vi "CheckListener ConvBox.vi"(8 "error in":errorcluster, 9 "address string":string, 11 "VISA resource in":refnum<visa-resource-name>) -> (0 "error out":errorcluster, 1 "listener found":bool, 2 "ibsta":T1, 3 "VISA resource out":refnum<visa-resource-name>)   [LabVIEW 2019, in "Protocols.lvlib" / "RS-xxx to GPIB ConvBox.lvclass"]
uses:
  RS-xxx to GPIB ConvBox.lvclass
  <vilib>/Instr/_visa.llb/GPIB Status Boolean Array.ctl
  <vilib>/Instr/_visa.llb/VISA Flush IO Buffer Mask.ctl
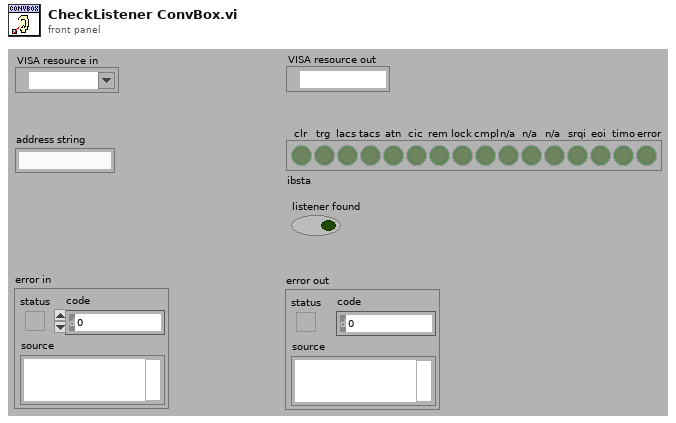
[diagram p1: front panel]
types:
  T1 = typedef "GPIB Status Boolean Array.ctl" = bool[]
  T2 = typedef "VISA Flush IO Buffer Mask.ctl" = u16
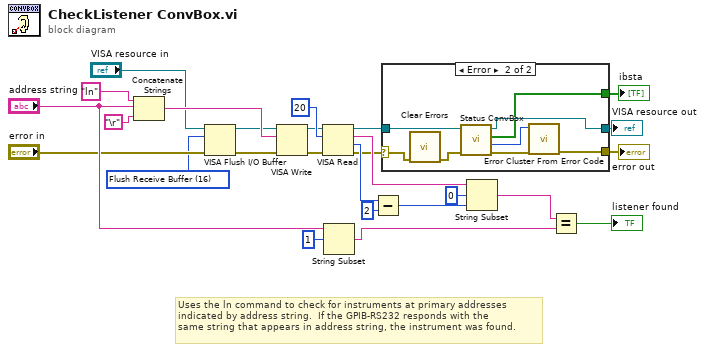
[diagram p0: block diagram]
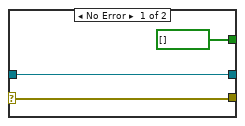
[diagram p2: hidden frame]
diagram:
  w6 = T2 16 items=["Flush Receive Buffer"=16, "Write Transmit Buffer to Device"=32, "Flush Receive Buffer (No I/O)"=64, "Flush Transmit Buffer"=128] ("Mask")
  # "Uses the ln command to check for instruments at primary addresses \nindicated by address string.  If the GPIB-RS232 responds with the\nsame string that appears in address string, the instrument was found."
  n1 = Concatenate Strings("ln", "address string", "\r") -> (w13:string)
  n2 = VISA Flush I/O Buffer(VISA resource name="VISA resource in", mask (16)=w6, error in (no error)="error in") -> (VISA resource name out=w9:refnum<visa-resource-name>, error out=w8:errorcluster)
  n3 = VISA Write(VISA resource name=w9, write buffer=w13, error in (no error)=w8) -> (VISA resource name out=w15:refnum<visa-resource-name>, error out=w14:errorcluster)  [unwired: 1 out]
  n4 = VISA Read(VISA resource name=w15, byte count=u32 20, error in (no error)=w14) -> (VISA resource name out=w5:refnum<visa-resource-name>, read buffer=w24:string, return count=w20:u32, error out=w4:errorcluster)
  n5 = String Subset(string="address string", offset (0)=1) -> (substring=w19:string)  [unwired: 1 in]
  n6 = Subtract(x=w20, y=u32 2) -> (x-y=w23:u32)
  n7 = case shown="Error" w4 {
    selector: w4 -> [w28 w30]
    tunnel: w5 -> [w29 w37]
    tunnel: [w28 w35] -> w3
    tunnel: [w29 w34] -> w2
    tunnel: [T1 [] ("ibsta") w32] -> w1
    frame No Error {
    }
    frame Error {
      n8 = call <vilib>:"Clear Errors.vi"("error in (no error)"=w30) -> ("error out"=w31:errorcluster)  [unwired: 5 in, 1 out]
      n9 = call "Status ConvBox.vi"("error in (no error)"=w31, "VISA resource name"=w37) -> ("error out"=w36:errorcluster, "GPIB error"=w33:i16, "ibsta"=w32:T1, "VISA resource out"=w34:refnum<visa-resource-name>)  [unwired: 6 in]
      n10 = call <vilib>:"Error Cluster From Error Code.vi"("error in (no error)"=w36, "error code (0)"=w33) -> ("error out"=w35:errorcluster)  [unwired: 7 in]
    }
  }
  "VISA resource out" <- w2
  "error out" <- w3
  "ibsta" <- w1
  n11 = String Subset(string=w24, offset (0)=0, length (rest)=w23) -> (substring=w25:string)
  n12 = Equal?(x=w25, y=w19) -> (x = y?=→"listener found":bool)
